vi "Set call to save ref.vi"(8 "error in":errorcluster, 11 "DAQCascade512II":refnum<class "DAQCascade512II.lvclass">) -> (0 "error out":errorcluster, 3 "DAQCascade512II out":refnum<class "DAQCascade512II.lvclass">)   [LabVIEW 2012, in "DAQCascade512II.lvclass"]
uses:
  DAQCascade512II.lvclass
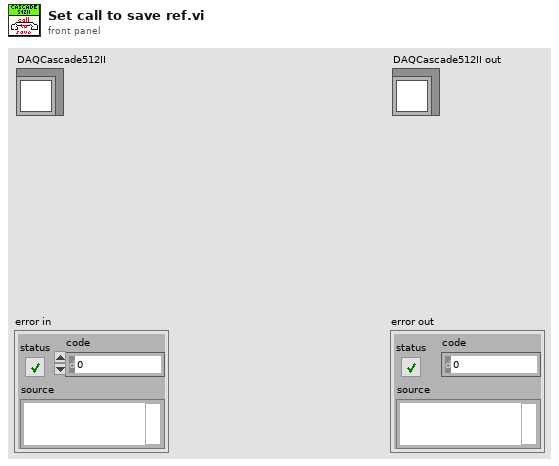
[diagram p1: front panel]
types:
  T1 = typedef "IMAQ Image.ctl" = refnum<image>
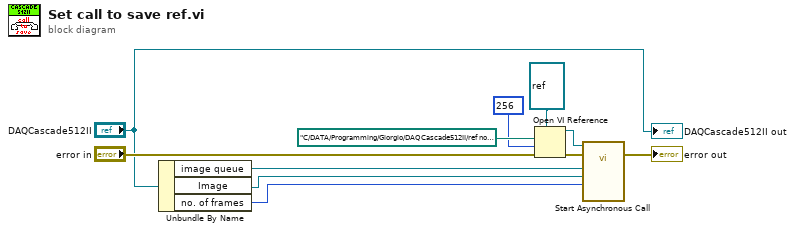
[diagram p0: block diagram]
diagram:
  n1 = Unbundle By Name("DAQCascade512II") -> ("image queue"=w3:refnum<queue>, "Image"=w2:T1, "no. of frames"=w1:u32)
  n2 = Open VI Reference(type specifier VI Refnum (for type only)=refnum<vi> refnum, vi path=path "C:/DATA/Programming/Giorgio/DAQCascade512II/ref nod test.vi", options=256, error in (no error)="error in") -> (vi reference=w10:refnum<vi>, error out=w9:errorcluster)  [unwired: 2 in]
  n3 = call-by-ref "Start Asynchronous Call"(reference=w10, error in=w9, "no. of frames"=w1, "Image"=w2, "image queue"=w3) -> (error out=→"error out":errorcluster)  [unwired: 8 in, 2 out]
  "DAQCascade512II out" <- "DAQCascade512II"
